vi "GetVersionNumberFromMutation.vi"(11 "Mutation History":T1 {"LabVIEW Version" format="%.0x"}) -> (2 "BlueSerializableVersion found?":bool, 3 "BlueSerializableVersion":u16)   [LabVIEW 2019, in "BlueSerializationProviderShared.lvlib"]
uses:
  BlueSerializationProviderShared.lvlib
  <vilib>/Utility/EditLVLibs/LVClass/Mutation History.ctl
  <vilib>/Utility/EditLVLibs/LVClass/Mutation Record.ctl
  <vilib>/Utility/EditLVLibs/LibVersion.ctl
  <vilib>/Utility/EditLVLibs/Edit LVLibs.lvlib
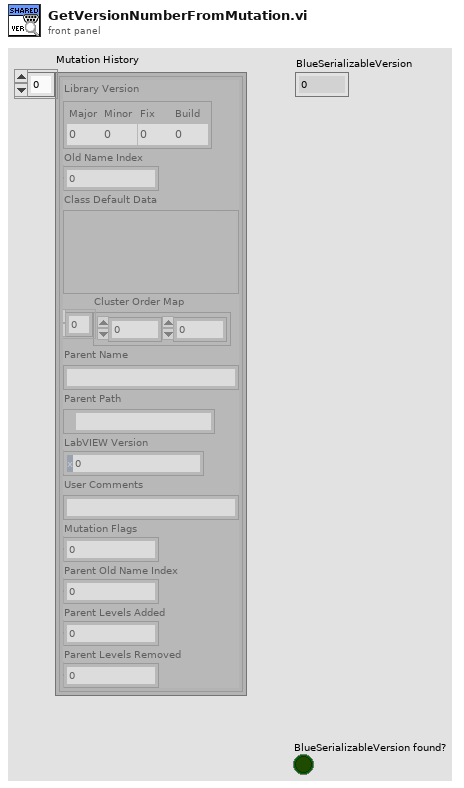
[diagram p1: front panel]
types:
  T1 = typedef "Edit LVLibs.lvlib/Mutation History.ctl" = T2[]
  T2 = typedef "Edit LVLibs.lvlib/Mutation Record.ctl" = cluster{"Library Version":T3, "Old Name Index":u8, "Class Default Data":variant, "Cluster Order Map":u32[], "Parent Name":string, "Parent Path":path, "LabVIEW Version":u32, "User Comments":string, "Mutation Flags":u8, "Parent Old Name Index":u8, "Parent Levels Added":u16, "Parent Levels Removed":u16}
  T3 = typedef "Edit LVLibs.lvlib/LibVersion.ctl" = cluster{"Major":u16, "Minor":u16, "Fix":u16, "Build":u16}
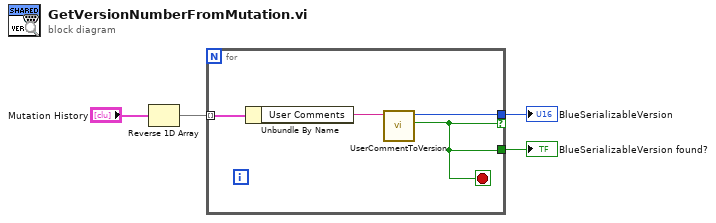
[diagram p0: block diagram]
diagram:
  n1 = Reverse 1D Array(array="Mutation History") -> (reversed array=w1:T1)
  n2 = for {
    tunnel: w1 -> [w8] mode=indexing
    tunnel: [w5] -> w4
    tunnel: [w6] -> w3 if=w5
    stop <- w5 stop-if-true
    n3 = Unbundle By Name(w8) -> ("User Comments"=w7:string)
    n4 = call "UserCommentToVersion.vi"("User Comment"=w7) -> ("BlueSerializableVersion found?"=w5:bool, "BlueSerializableVersion"=w6:u16)  [unwired: 9 in]
  }
  "BlueSerializableVersion found?" <- w4
  "BlueSerializableVersion" <- w3
